vi "Create.vi"(8 "error in (no error)":errorcluster) -> (0 "error out":errorcluster, 3 "mqttCmdPingResponse out":refnum<class "PingResponseMqttMsg.lvclass">)   [LabVIEW 2020, in "PingResponseMqttMsg.lvclass"]
uses:
  PingResponseMqttMsg.lvclass
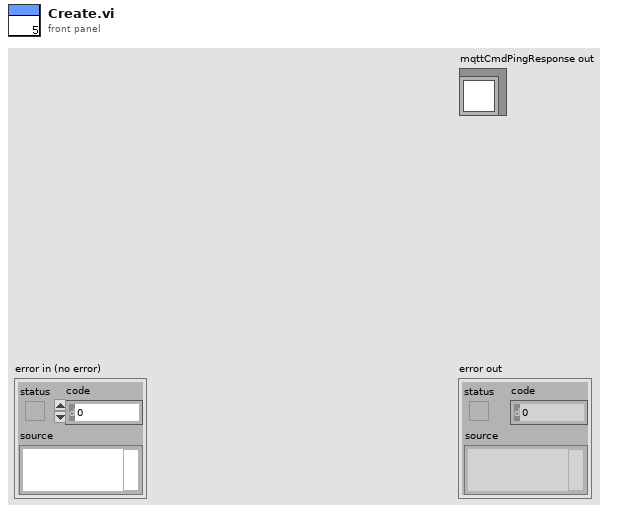
[diagram p1: front panel]
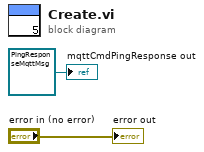
[diagram p0: block diagram]
diagram:
  "error out" <- "error in (no error)"
  "mqttCmdPingResponse out" <- refnum<class "PingResponseMqttMsg.lvclass"> refnum ("mqttCmdPingResponse in")
